vi "Robot Centric.vi"(0 "X Axis":dbl, 3 "Tracks Down":bool, 4 "Drive 1":string="RobotDrive", 5 "Y Axis":dbl, 7 "Z Axis":dbl) -> ()   [LabVIEW 2018]
uses:
  <vilib>/Rock Robotics/WPI/Utilities/WPI_GetSetVariantRefNum.vi
  <vilib>/Rock Robotics/WPI/RobotDrive/WPI_RobotDriveMecanumDrive_Cartesian.vi
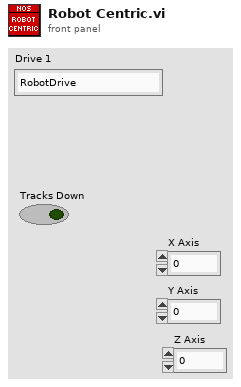
[diagram p1: front panel]
types:
  T1 = typedef "WPI_RobotDriveDevRef.ctl" = cluster{"DevStatus":errorcluster, "Motors[]":T2[], "Square Inputs":bool, "Max Output":dbl}
  T2 = typedef "WPI_MotorControlDeviceRef.ctl" = cluster{"DeviceStatus":errorcluster, "Type":T3, "PWM":cluster{"PWM Channel":T4, "DeadBand":T5}, "CAN":cluster{"Device Number":u8, "SetOutput VI Ref":variant, "GetOutput VI Ref":variant, "Enable VI Ref":variant, "Disable VI Ref":variant, "Data":variant}, "Invert":bool, "DIO PWM":cluster{"PWM \"Enable\" Channel":T4, "DIOChannel":T6, "PWM Rate":dbl}}
  T3 = typedef "WPI_MotorControlType.ctl" = enum16{"PWM", "CAN", "DIO PWM"}
  T4 = typedef "FPGA_DIOPWMChannel.ctl" = enum8{"PWM 0", "PWM 1", "PWM 2", "PWM 3", "PWM 4", "PWM 5", "PWM 6", "PWM 7", "PWM 8", "PWM 9", "PWM MXP 0", "PWM MXP 1", "PWM MXP 2", "PWM MXP 3", "PWM MXP 4", "PWM MXP 5", "PWM MXP 6", "PWM MXP 7", "PWM MXP 8", "PWM MXP 9", "Invalid"}
  T5 = typedef "WPI_PWMDeadband.ctl" = cluster{"Name":string, "maxPositivePwm":i32, "minPositivePwm":i32, "centerPwm":i32, "maxNegativePwm":i32, "minNegativePwm":i32, "angularRange":u16}
  T6 = typedef "FPGA_DIOChannel.ctl" = enum8{"DIO 0", "DIO 1", "DIO 2", "DIO 3", "DIO 4", "DIO 5", "DIO 6", "DIO 7", "DIO 8", "DIO 9", "DIO MXP 0", "DIO MXP 1", "DIO MXP 2", "DIO MXP 3", "DIO MXP 4", "DIO MXP 5", "DIO MXP 6", "DIO MXP 7", "DIO MXP 8", "DIO MXP 9", "DIO MXP 10", "DIO MXP 11", "DIO MXP 12", "DIO MXP 13", "DIO MXP 14", "DIO MXP 15", "SPI Port CS1", "SPI Port CS2", "SPI Port CS3", "SPI Port MISO", "SPI Port MOSI", "Invalid"}
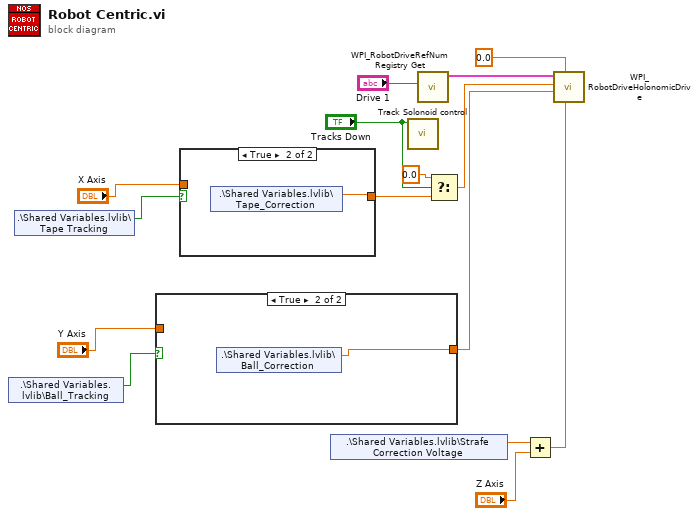
[diagram p0: block diagram]
diagram:
  n1 = shared-variable ".\\Shared Variables.lvlib\\Ball_Tracking"() -> (w1:bool)  [unwired: 1 in, 1 out]
  n2 = shared-variable ".\\Shared Variables.lvlib\\Tape Tracking"() -> (w4:bool)  [unwired: 1 in, 1 out]
  n3 = case shown="True" w1 {
    tunnel: [w16 w17] -> w3
    tunnel: "Y Axis" -> [w16 _]
    frame False {
    }
    frame True {
      n4 = shared-variable ".\\Shared Variables.lvlib\\Ball_Correction"() -> (w17:dbl)  [unwired: 1 in, 1 out]
    }
  }
  n5 = case shown="True" w4 {
    tunnel: [w18 w19] -> w6
    tunnel: "X Axis" -> [w18 _]
    frame False {
    }
    frame True {
      n6 = shared-variable ".\\Shared Variables.lvlib\\Tape_Correction"() -> (w19:dbl)  [unwired: 1 in, 1 out]
    }
  }
  n7 = shared-variable ".\\Shared Variables.lvlib\\Strafe Correction Voltage"() -> (w7:dbl)  [unwired: 1 in, 1 out]
  n8 = call "Track Solonoid control.vi"("Manual Tracks"="Tracks Down") -> ()  [unwired: 11 in]
  n9 = call <vilib>:"WPI_RobotDriveRefNum Registry Get.vi"("refnum name"="Drive 1") -> ("RobotDriveDevRef"=w10:T1)  [unwired: 9 in, 1 out]
  n10 = Select(t=0.0, s="Tracks Down", f=w6) -> (s? t:f=w11:dbl)
  n11 = Add(x=w7, y="Z Axis") -> (x+y=w13:dbl)
  n12 = call-poly <vilib>:"WPI_RobotDriveHolonomicDrive.vi"("Rotation"=w13, "Gyro Angle"=0.0, "Y"=w3, "X"=w11, "RobotDriveDevRef"=w10) -> ()  [unwired: 4 in, 3 out]
